vi "Dlg-Edit-Exchanges.vi"(8 "error in (no error)":errorcluster, 9 "Parameters":T1, 10 "Key":i32, 11 "Exchanges in":refnum<class "Exchanges.lvclass">) -> (0 "error out":errorcluster, 2 "Canceled":bool, 3 "Exchanges out":refnum<class "Exchanges.lvclass">)   [LabVIEW 2012]
uses:
  controls/Currencies.ctl
  Exchanges.lvclass
  Exchange/Exchange Type Enum.ctl
  Exchange/Exchange Parameters.ctl
  Stock/Stock.lvclass/Stock.ctl
  Exchange/Exchange.lvclass
  Stock/Stock.lvclass
panel:
  in  "Search Stock":bool
  out "Label":string
  out "ISIN":string
  in  "Taxe":dbl
  in  "Quantité":dbl
  in  "Type":T2
  in  "Currency":T3
  in  "Prix":dbl
  in  "Edit":bool
  in  "Date":timestamp format="%<%X\n%x>T"
  in  "Commentaires":string
  in  "Cancel Button":bool
  in  "Help":bool
  # "Nouveau Portefeuille"
  # "Editer une Transaction"
  # "Transaction"
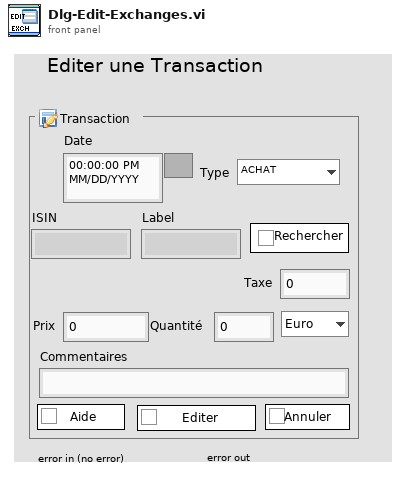
[diagram p1: front panel]
types:
  T1 = typedef "Exchange Parameters.ctl" = cluster{"Date":timestamp, "Exchange Type":T2, "ISIN":string, "Label":string, "Price":dbl, "Qty":dbl, "Currency":T3, "Tax":dbl, "Comment":string, "PRU":dbl}
  T2 = typedef "Exchange.lvclass/Exchange Type Enum.ctl" = enum16{"ACHAT", "VENTE"}
  T3 = typedef "Currencies.ctl" = enum16{"Euro", "Dollar", "Yen", "RIM", "CHF"}
  T4 = enum8{"Enabled", "Disabled", "Disabled and Grayed Out"}
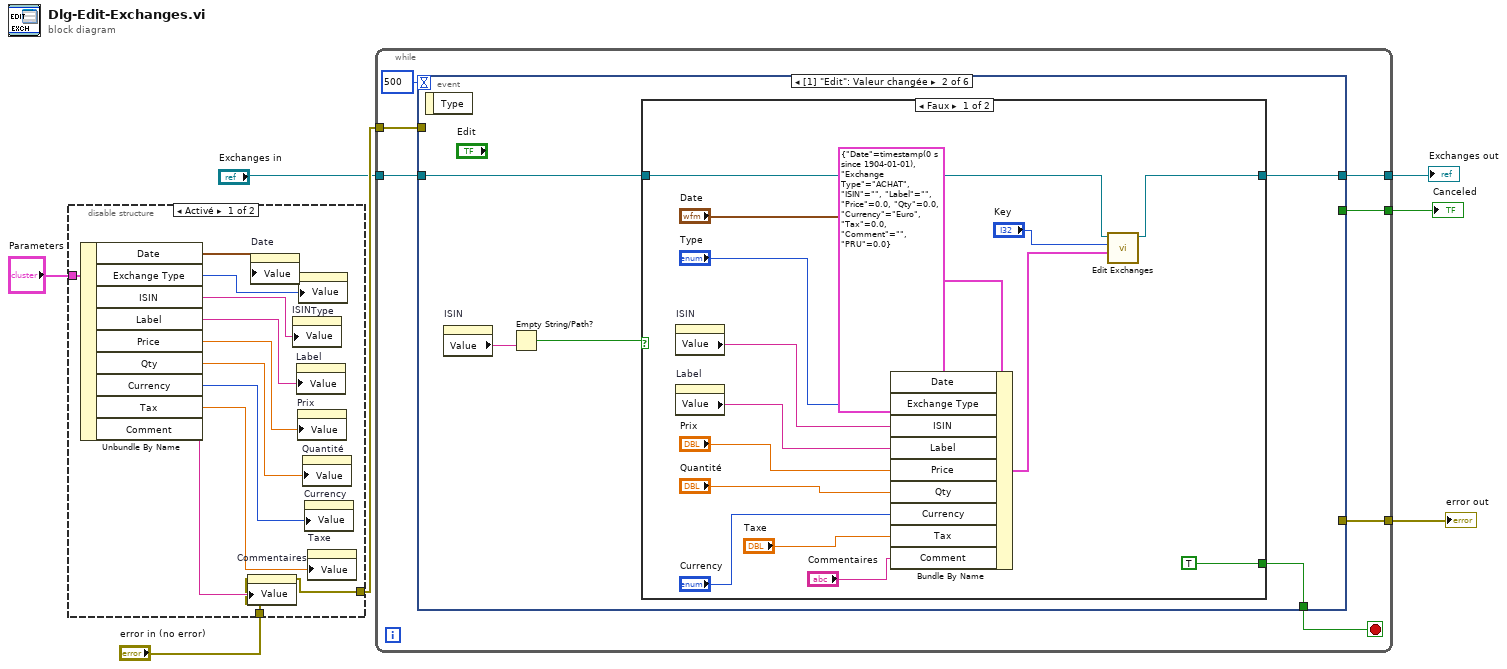
[diagram p0: block diagram]
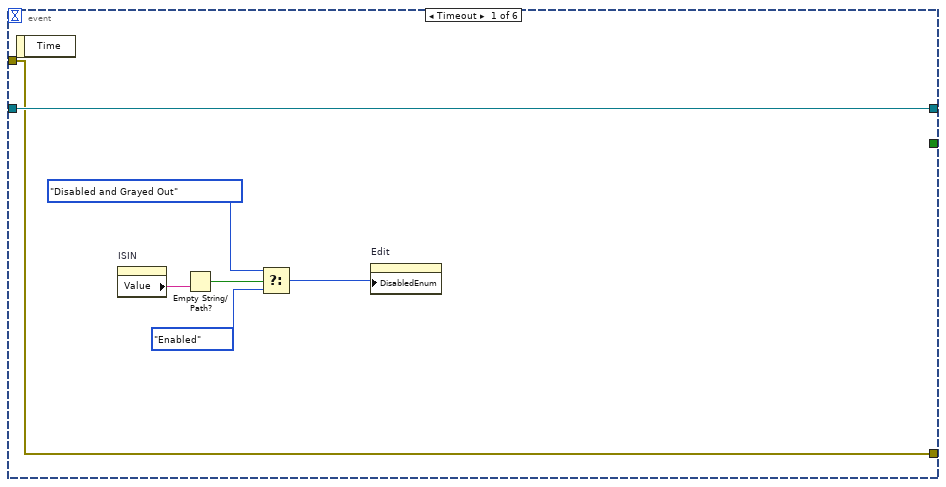
[diagram p2: hidden frame]
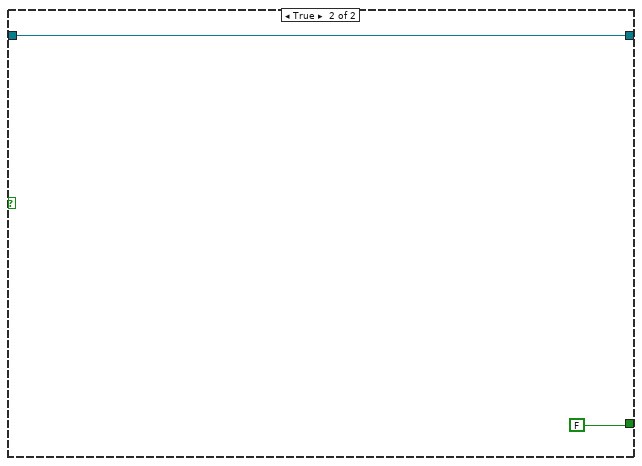
[diagram p3: hidden frame]
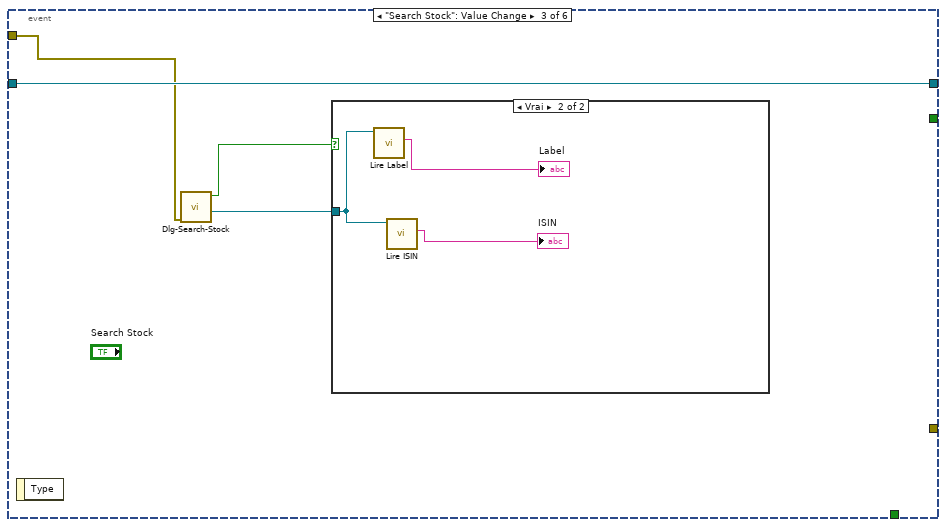
[diagram p4: hidden frame]
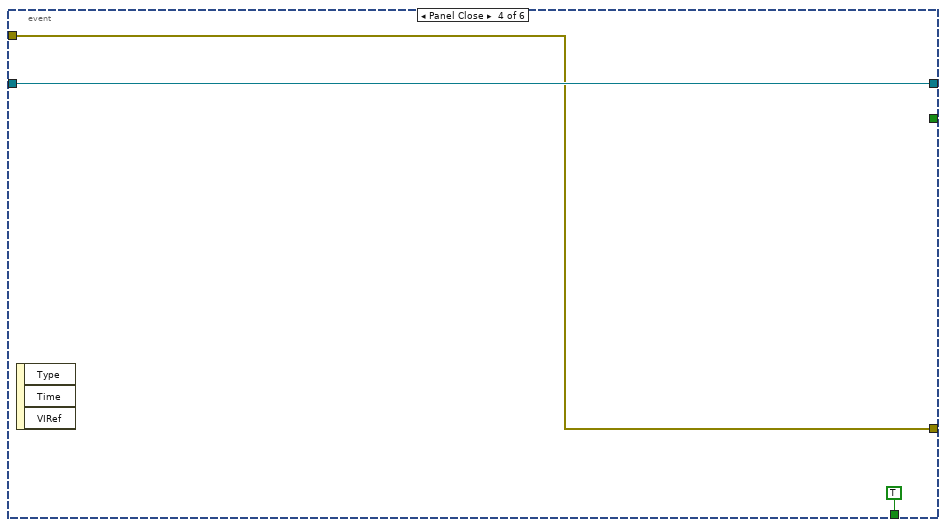
[diagram p6: hidden frame]
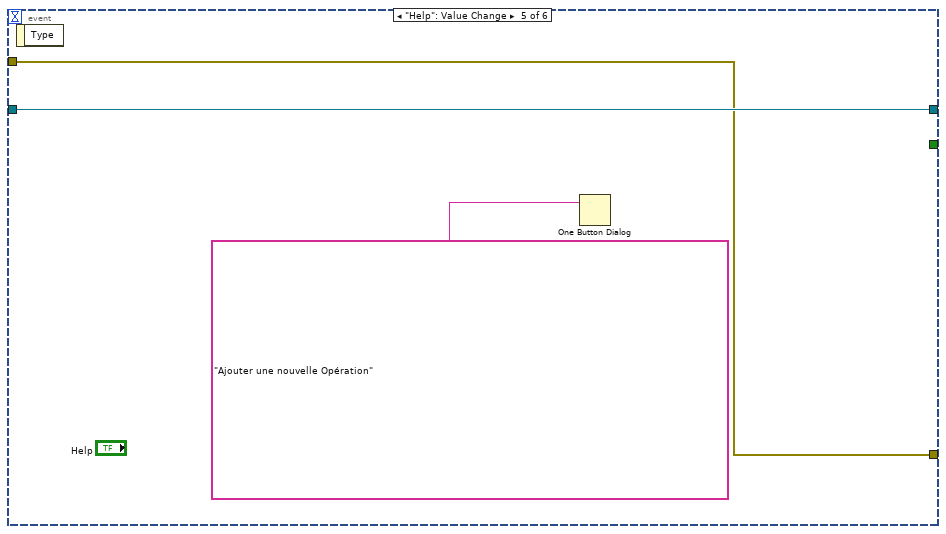
[diagram p7: hidden frame]
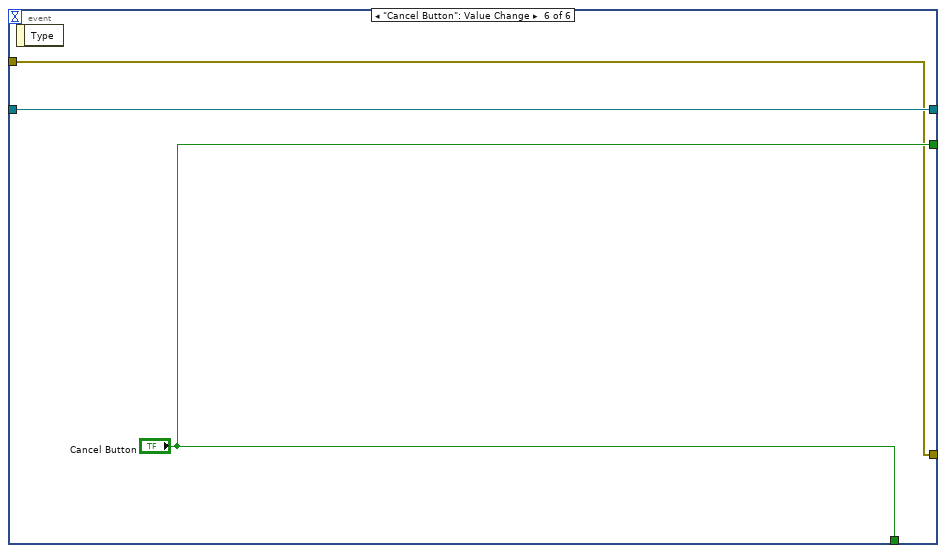
[diagram p8: hidden frame]
diagram:
  n1 = disable-structure shown="Activé" {
    disable-tunnel: [w8 _] -> w7
    disable-tunnel: "error in (no error)" -> [w9 _]
    disable-tunnel: "Parameters" -> [w19 _]
    frame Enabled {
      n2 = Unbundle By Name(w19) -> ("Date"=w18:timestamp, "Exchange Type"=w17:T2, "ISIN"=w16:string, "Label"=w15:string, "Price"=w14:dbl, "Qty"=w13:dbl, "Currency"=w12:T3, "Tax"=w11:dbl, "Comment"=w10:string)
      n3 = property on="Commentaires" class="Ch"(error in=w9, "Value"=w10) -> (error out=w8:errorcluster)  [unwired: 1 in, 1 out]
      n4 = property on="Date" class="TempsAbs (strict)"("Value"=w18) -> ()  [unwired: 2 in, 2 out]
      n5 = property on="ISIN" class="Ch"("Value"=w16) -> ()  [unwired: 2 in, 2 out]
      n6 = property on="Label" class="Ch"("Value"=w15) -> ()  [unwired: 2 in, 2 out]
      n7 = property on="Prix" class="NumNb (strict)"("Value"=w14) -> ()  [unwired: 2 in, 2 out]
      n8 = property on="Type" class="Énum (strict)"("Value"=w17) -> ()  [unwired: 2 in, 2 out]
      n9 = property on="Quantité" class="NumNb (strict)"("Value"=w13) -> ()  [unwired: 2 in, 2 out]
      n10 = property on="Currency" class="Énum (strict)"("Value"=w12) -> ()  [unwired: 2 in, 2 out]
      n11 = property on="Taxe" class="NumNb (strict)"("Value"=w11) -> ()  [unwired: 2 in, 2 out]
    }
    frame Disabled {
    }
  }
  n12 = while {
    tunnel: w7 -> [w26]
    tunnel: [w25] -> w5
    tunnel: "Exchanges in" -> [w24]
    tunnel: [w23] -> w3
    tunnel: [w21] -> w2
    stop <- w22 stop-if-true
    n13 = event shown="[1] \"Edit\": Valeur changée" {
      selector: _ -> [_ _ _ _ _ _]
      dyn-events: _ -> [_ _ _ _ _ _]
      timeout: 500 -> [_ _ _ _ _ _]
      tunnel: w26 -> [w32 _ w58 w63 w66 w69]
      tunnel: [_ _ _ _ _ "Cancel Button"] -> w25
      tunnel: w24 -> [w33 w38 w59 w64 w67 w71]
      tunnel: [w33 w37 w59 w64 w67 w71] -> w23
      tunnel: [_ w34 _ TRUE ("Cancel Button") _ "Cancel Button"] -> w22
      tunnel: [w32 _ _ w63 w66 w69] -> w21
      event Timeout {
        n14 = event-data() -> ()  [unwired: 1 in, 1 out]
        n15 = property on="ISIN" class="Ch"() -> ("Value"=w31:string)  [unwired: 2 in, 2 out]
        n16 = Empty String/Path?(string/path=w31) -> (empty?=w30:bool)
        n17 = Select(t=T4."Disabled and Grayed Out" ("Désactivé"), s=w30, f=T4."Enabled" ("Désactivé")) -> (s? t:f=w28:T4)
        n18 = property on="Edit" class="Bool"("DisabledEnum"=w28) -> ()  [unwired: 2 in, 2 out]
      }
      event "Edit": Value Change {
        n19 = event-data() -> ()  [unwired: 1 in, 1 out]
        n20 = property on="ISIN" class="Ch"() -> ("Value"=w36:string)  [unwired: 2 in, 2 out]
        n21 = Empty String/Path?(string/path=w36) -> (empty?=w35:bool)
        n22 = case shown="Faux" w35 {
          tunnel: w38 -> [w52 w55]
          tunnel: [w51 w55] -> w37
          tunnel: [TRUE ("vide ?") FALSE ("vide ?")] -> w34
          frame False {
            n23 = property on="ISIN" class="Ch"() -> ("Value"=w43:string)  [unwired: 2 in, 2 out]
            n24 = property on="Label" class="Ch"() -> ("Value"=w42:string)  [unwired: 2 in, 2 out]
            n25 = Bundle By Name(cluster=T1 {"Date"=timestamp(0 s since 1904-01-01), "Exchange Type"=enum."ACHAT", "ISIN"="", "Label"="", "Price"=0.0, "Qty"=0.0, "Currency"=enum."Euro", "Tax"=0.0, "Comment"="", "PRU"=0.0} ("Parameters"), "Date"="Date", "Exchange Type"="Type", "ISIN"=w43, "Label"=w42, "Price"="Prix", "Qty"="Quantité", "Currency"="Currency", "Tax"="Taxe", "Comment"="Commentaires") -> (w40:T1)
            n26 = call "Edit Exchanges.vi"("Parameters"=w40, "Key"="Key", "Exchanges en entrée"=w52) -> ("Exchanges en sortie"=w51:refnum<class "Exchanges.lvclass">)  [unwired: 6 in, 2 out]
          }
          frame True {
          }
        }
      }
      event "Search Stock": Value Change {
        n27 = event-data() -> ()  [unwired: 1 in, 1 out]
        n28 = call "Dlg-Search-Stock.vi"("error in (no error)"=w58) -> ("Stock Selected"=w56:refnum<class "Stock.lvclass">, "OK ?"=w57:bool)  [unwired: 7 in, 2 out]
        n29 = case shown="Vrai" w57 {
          tunnel: w56 -> [_ w62]
          frame False {
          }
          frame True {
            n30 = call "Lire Label.vi"("Share en entrée"=w62) -> ("Label"=→"Label":string)  [unwired: 8 in, 2 out]
            n31 = call "Lire ISIN.vi"("Share en entrée"=w62) -> ("ISIN"=→"ISIN":string)  [unwired: 8 in, 2 out]
          }
        }
      }
      event Panel Close {
        n32 = event-data() -> ()  [unwired: 1 in, 3 out]
      }
      event "Help": Value Change {
        n33 = event-data() -> ()  [unwired: 1 in, 1 out]
        n34 = One Button Dialog(message="Ajouter une nouvelle Opération") -> ()  [unwired: 1 in, 1 out]
      }
      event "Cancel Button": Value Change {
        n35 = event-data() -> ()  [unwired: 1 in, 1 out]
      }
    }
  }
  "error out" <- w2
  "Canceled" <- w5
  "Exchanges out" <- w3
